vi "RSNRPZ Get Scope Measurements Level Thresholds.vi"(8 "error in (no error)":errorcluster, 10 "Channel (1)":i32=1, 11 "VISA session":refnum<visa-resource-name> caption="VISA resource name") -> (0 "error out":errorcluster, 1 "Duration Ref":dbl format="%^.3e", 3 "dup VISA session":refnum<visa-resource-name> caption="VISA resource name", 4 "Transition Low Ref":dbl format="%^.3e", 5 "Transition High Ref":dbl format="%^.3e")   [LabVIEW 2010]
doc: "This VI queries the thresholds of the reference and transition levels that are used for the calculation of the pulse's time parameter.\n\nNote:\n1) This VI is only available for NRP-Z81.\n\nRemote-control command(s):\nSENS:TRAC:MEAS:DEF:DUR:REF? \nSENS:TRAC:MEAS:DEF:TRAN:LREF?\nSENS:TRAC:MEAS:DEF:TRAN:HREF?"
uses:
  rsnrpz_32.dll
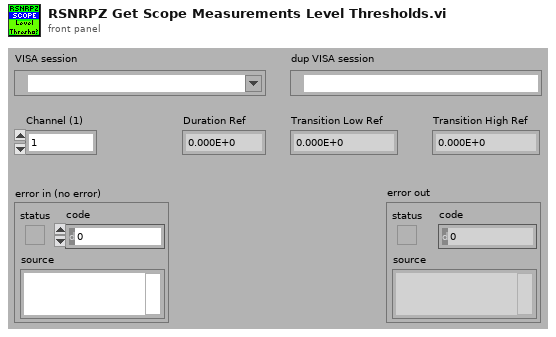
[diagram p1: front panel]
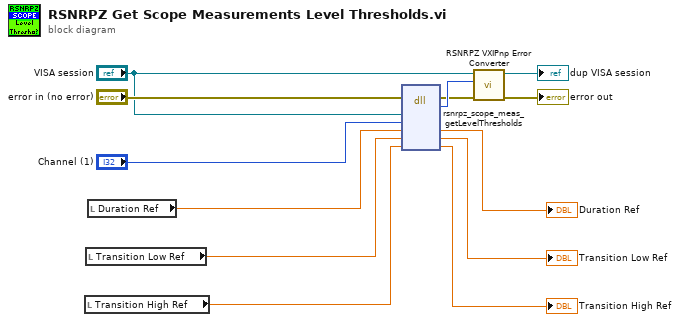
[diagram p0: block diagram]
diagram:
  n1 = local read "Transition High Ref"() -> (w7:dbl)
  n2 = local read "Transition Low Ref"() -> (w9:dbl)
  n3 = local read "Duration Ref"() -> (w11:dbl)
  n4 = dll-call lib="rsnrpz_32.dll" fn="rsnrpz_scope_meas_getLevelThresholds"(error in="error in (no error)", "Instrument Handle"="VISA session", "Channel"="Channel (1)", "Duration Ref"=w11, "Transition Low Ref"=w9, "Transition High Ref"=w7) -> (error out=w5:errorcluster, "Status"=w13:i32, "Duration Ref"=→"Duration Ref":dbl, "Transition Low Ref"=→"Transition Low Ref":dbl, "Transition High Ref"=→"Transition High Ref":dbl)  [unwired: 4 in, 1 out]
  n5 = call <instrlib>:"RSNRPZ VXIPnp Error Converter.vi"("error in"=w5, "VXIPnp error code"=w13, "VISA session"="VISA session") -> ("error out"=→"error out":errorcluster, "dup VISA session"=→"dup VISA session":refnum<visa-resource-name>)  [unwired: 7 in]
